vi "Read Async.vi"(7 "NumberOfBuffers":u32, 8 "error in (no error)":errorcluster, 9 "BufferLength":u32, 10 "user event out":refnum<user-event>, 11 "DeviceRefnum":u64) -> (0 "error out":errorcluster, 2 "function return":i32, 3 "DeviceRefnum Out":u64)   [LabVIEW 2016]
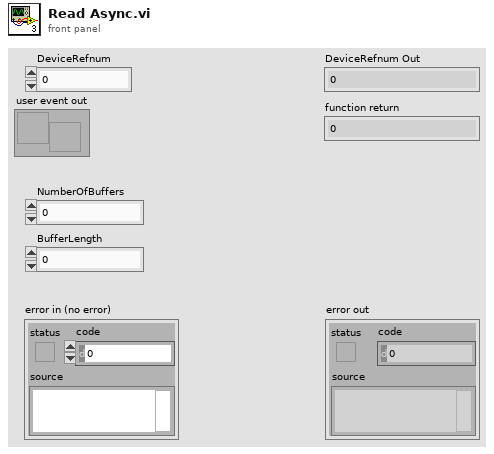
[diagram p1: front panel]
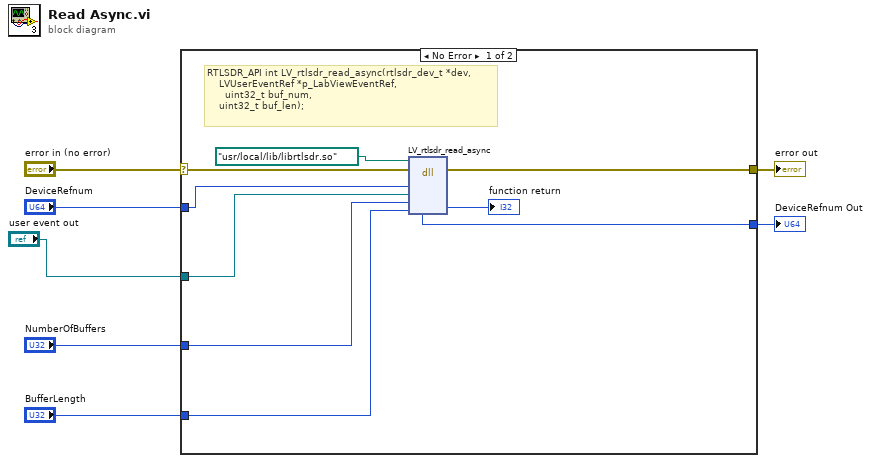
[diagram p0: block diagram]
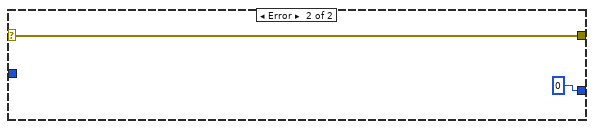
[diagram p2: hidden frame]
diagram:
  n1 = case shown="No Error" "error in (no error)" {
    selector: "error in (no error)" -> [w12 w18]
    tunnel: [w15 w18] -> w7
    tunnel: [w14 u64 0 ("DeviceRefnum")] -> w6
    tunnel: "DeviceRefnum" -> [w11 _]
    tunnel: "user event out" -> [w10 _]
    tunnel: "NumberOfBuffers" -> [w9 _]
    tunnel: "BufferLength" -> [w8 _]
    frame No Error {
      # "RTLSDR_API int LV_rtlsdr_read_async(rtlsdr_dev_t *dev, \n\t\t\t\tLVUserEventRef *p_LabViewEventRef, \n\t\t\t  \tuint32_t buf_num, \n\t\t\t\tuint32_t buf_len);"
      n2 = dll-call lib="usr/local/lib/librtlsdr.so" fn="LV_rtlsdr_read_async"(path in=path "/usr/local/lib/librtlsdr.so", error in=w12, "DeviceRefnum"=w11, "LVUserEventRef"=w10, "NumberOfBuffers"=w9, "BufferLength"=w8) -> (error out=w15:errorcluster, "return type"=→"function return":i32, "DeviceRefnum"=w14:u64)  [unwired: 4 in, 1 out]
    }
    frame Error {
    }
  }
  "error out" <- w7
  "DeviceRefnum Out" <- w6
